vi "Configure Polynomial Calculation.vi"(7 "a2 Factor (0.000000E+0)":dbl format="%.6e", 8 "error in (no error)":errorcluster, 9 "a1 Factor (1.000000E+0)":dbl=1.0 format="%.6e", 10 "a0 Factor (0.000000E+0)":dbl format="%.6e", 11 "VISA resource name":refnum<visa-resource-name>) -> (0 "error out":errorcluster, 3 "VISA resource name out":refnum<visa-resource-name>)   [LabVIEW 2020, in "Keithley 6517.lvlib"]
doc: "Configures the \"a0\", \"a1\" and \"a2\" factor for the polynomial calculation.\n\n<B>Note:</B>\nThis VI is <B>NOT</B> compatible with model <B>6514</B>."
uses:
  <instrlib>/Keithley 6517/Keithley 6517.lvlib
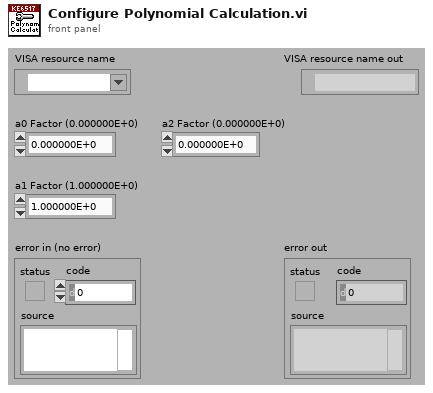
[diagram p1: front panel]
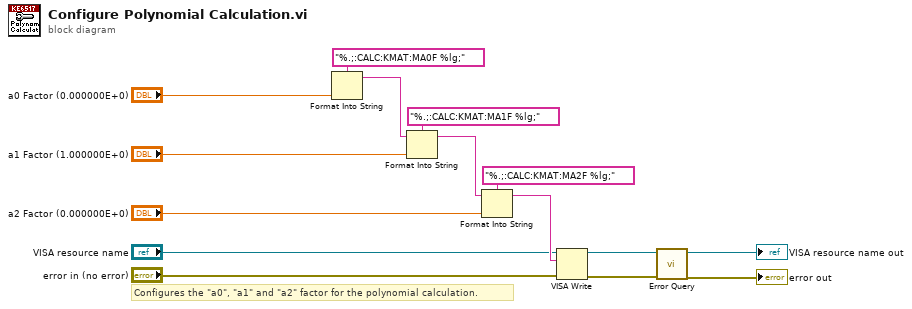
[diagram p0: block diagram]
diagram:
  # "Configures the \"a0\", \"a1\" and \"a2\" factor for the polynomial calculation."
  n1 = Format Into String(format string="%.;:CALC:KMAT:MA0F %lg;", "a0 Factor (0.000000E+0)") -> (resulting string=w13:string)  [unwired: 2 in, 1 out]
  n2 = Format Into String(format string="%.;:CALC:KMAT:MA1F %lg;", initial string=w13, "a1 Factor (1.000000E+0)") -> (resulting string=w10:string)  [unwired: 1 in, 1 out]
  n3 = Format Into String(format string="%.;:CALC:KMAT:MA2F %lg;", initial string=w10, "a2 Factor (0.000000E+0)") -> (resulting string=w7:string)  [unwired: 1 in, 1 out]
  n4 = VISA Write(VISA resource name="VISA resource name", write buffer=w7, error in (no error)="error in (no error)") -> (VISA resource name out=w5:refnum<visa-resource-name>, error out=w4:errorcluster)  [unwired: 1 out]
  n5 = call <instrlib>:"Error Query.vi"("error in (no error)"=w4, "VISA resource name"=w5) -> ("error out"=→"error out":errorcluster, "VISA resource name out"=→"VISA resource name out":refnum<visa-resource-name>)  [unwired: 6 in, 2 out]
